vi "Write Speed [km_h].vi"(8 "error in (no error)":errorcluster, 10 "Speed [km/h]":dbl, 11 "Spaceship in":refnum<class "Spaceship.lvclass">) -> (0 "error out":errorcluster, 3 "Spaceship out":refnum<class "Spaceship.lvclass">)   [LabVIEW 2021, in "Spaceship.lvclass"]
uses:
  Spaceship.lvclass
  Spaceship.lvclass/Spaceship.ctl
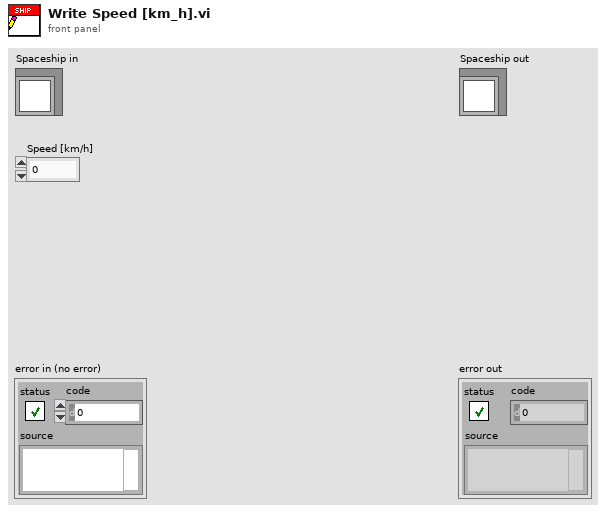
[diagram p1: front panel]
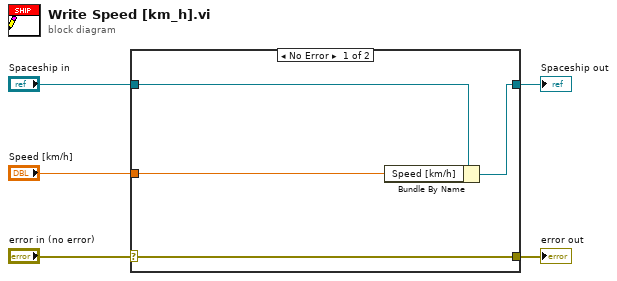
[diagram p0: block diagram]
diagram:
  n1 = case shown="No Error" "error in (no error)" {
    selector: "error in (no error)" -> [w9 w10]
    tunnel: [w9 w10] -> w4
    tunnel: [w7 w11] -> w2
    tunnel: "Spaceship in" -> [w8 w11]
    tunnel: "Speed [km/h]" -> [w6 _]
    frame No Error {
      n2 = Bundle By Name(cluster=w8, "Speed [km/h]"=w6) -> (w7:refnum<class "Spaceship.lvclass">)
    }
    frame Error {
    }
  }
  "error out" <- w4
  "Spaceship out" <- w2
